vi "Intellirupter_main.vi"() -> ()   [LabVIEW 2016]
uses:
  <vilib>/Platform/TimedLoop/XDataNode/timing_clust.ctl
  <vilib>/Platform/TimedLoop/XDataNode/nitl_modes.ctl
  <vilib>/Platform/TimedLoop/XDataNode/wakeup.ctl
  <vilib>/FPGAPlugInAG/cRIO-9039 (Sync)/niLvFpga_Open_cRIO-9039 (Sync).vi
  <vilib>/rvi/interface/common/dynamic/niFpgaDynamicAddResources.vi
  <vilib>/Utility/error.llb/Error Cluster From Error Code.vi
  <vilib>/rvi/errors/niLvFpgaAdjustHostInterfaceError.vi
  Communication (Yiwei)/Global communication.vi
  <vilib>/FPGAPlugInAG/Dynamic/niLvFpga_Close_Dynamic.vi
  <vilib>/rvi/interface/nirviOpenFPGA/nirviOpenFPGA.xnode
  FPGA Bitfiles/IntelliRupter_calibrated.lvbitx
  <vilib>/rvi/interface/nirviReadWriteControl/nirviReadWriteControl.xnode
  <vilib>/Platform/TimedLoop/XDataNode/XDataNode.xnode
  <vilib>/rvi/interface/nirviCloseFPGA/nirviCloseFPGA.xnode
  <vilib>/rvi/interface/Simulation/niFpgaSimulationCallBeginRW.vi
  NiFpgaLv.dll
  <vilib>/Platform/TimedLoop/XDataNode/XDNodeRunTimeDep.lvlib
panel:
  out "Waveform Chart 2":dbl(graph)
  in  "output cluster":cluster{"reinitialize? (F)":bool, "dt (s)":dbl}={"reinitialize? (F)"=FALSE, "dt (s)"=0.001}
  in  "PID gains":T1={"proportional gain (Kc)"=1.0, "integral time (Ti, min)"=0.001, "derivative time (Td, min)"=0.0} {"derivative time (Td, min)" format="%.3f"; "integral time (Ti, min)" format="%.3f"; "proportional gain (Kc)" format="%.3f"}
  in  "y":dbl
  out "Waveform Chart":dbl(graph)
  in  "I offset R2":dbl=-0.06
  in  "I offset R7":dbl
  in  "I offset R3":dbl=-0.12
  out "R8 Transfer":bool
  out "R7 Transfer":bool
  out "R5 Transfer":bool
  out "R4 Transfer":bool
  out "R2 Transfer":bool
  in  "I offset R8":dbl=0.09
  in  "I offset R4":dbl=-0.07
  in  "I offset R6":dbl=0.095
  in  "I offset R5":dbl=0.02
  in  "I offset R1":dbl=-0.12
  in  "R8 Blocking in":bool
  in  "R7 Blocking in":bool
  in  "R6 Blocking in":bool
  in  "R5 Blocking in":bool
  in  "R4 Blocking in":bool
  in  "R3 Blocking in":bool
  in  "R2 Blocking in":bool
  in  "R1 Blocking in":bool
  out "R1 Blocking out":bool[](array[boolean])
  out "R2 Blocking out":bool[](array[boolean])
  out "R3 Blocking out":bool[](array[boolean])
  out "R4 Blocking out":bool[](array[boolean])
  out "R5 Blocking out":bool[](array[boolean])
  out "R6 Blocking out":bool[](array[boolean])
  out "R8 Blocking out":bool[](array[boolean])
  out "R7 Blocking out":bool[](array[boolean])
  out "Relay7 Reclose":bool=TRUE
  out "Relay7 Trip":bool
  out "Relay8 Reclose":bool=TRUE
  out "Relay8 Trip":bool
  out "Relay6 Reclose":bool=TRUE
  out "Relay6 Trip":bool
  out "Relay5 Reclose":bool=TRUE
  out "Relay5 Trip":bool
  out "Relay4 Reclose":bool=TRUE
  out "Relay4 Trip":bool
  out "Relay3 Reclose":bool=TRUE
  out "Relay3 Trip":bool
  out "Relay2 Reclose":bool=TRUE
  out "Relay2 Trip":bool
  out "Relay1 Reclose":bool=TRUE
  out "Relay1 Trip":bool
  in  "Manual Relay Control":bool
  in  "Reset Relay":bool
  out "Loop time":u32=37
  in  "Recloser Settings":T2={"Magnitude Minimum"=0.1, "Magnitude difference level"=0.1, "Frequency difference level"=0.5, "Phase difference level"=10.0}
  out "MGCC_to_relay":bool[](array[boolean])=[TRUE, TRUE, FALSE, TRUE, TRUE, TRUE, TRUE, TRUE]
  in  "Count(ticks)":u32=10000
  in  "RMS minimum\nvalues":cluster{"VRMS values":dbl, "IRMS values":dbl}={"VRMS values"=0.1, "IRMS values"=0.1}
  out "error out":errorcluster
  out "Relay_toMGCC":bool[](array[boolean])=[TRUE, TRUE, FALSE, TRUE, TRUE, TRUE, TRUE, TRUE]
  in  "Reclose Relay8?":bool=TRUE
  out "R8 Data for\ncommunication":dbl[](array[numeric])=[1.0, 1.0717288119606128, 1.0273744109493954, 60.14375742781454, 60.14096390508348, -0.003401189111173153, 0.13142361409120604, 0.0014423221455373873, 0.0, 0.0]
  in  "Reclose Relay7?":bool=TRUE
  out "R7 Data for\ncommunication":dbl[](array[numeric])=[1.0, 1.0189736883003988, 1.0391105774878193, 60.14220400137767, 60.14841362237464, -0.003401275025680661, -0.31916486626176716, -0.003154578866978825, 0.0, 0.0]
  in  "Reclose Relay6?":bool=TRUE
  out "R6 Data for\ncommunication":dbl[](array[numeric])=[1.0, 1.1139535808581806, 1.0329364281545637, 60.147215439773106, 60.14857986423551, -0.003401093650609255, 0.12186050090227488, -0.001429571057703036, 0.0, 0.0]
  in  "Reclose Relay5?":bool=TRUE
  out "R5 Data for\ncommunication":dbl[](array[numeric])=[1.0, 1.1121379065253558, 1.0317589511765997, 60.14737789614628, 60.15040153111249, -0.0034011360257864, -0.20946315978329266, -0.0021582839957721063, 0.0, 0.0]
  in  "Reclose Relay4?":bool=TRUE
  out "R4 Data for\ncommunication":dbl[](array[numeric])=[1.0, 1.0686115234679994, 1.0027287608315838, 60.152969027967806, 60.13754923755685, -0.0034010736271739006, -0.14980308382633703, 0.0013760159412812356, 0.0, 0.0]
  in  "Reclose Relay3?":bool
  out "R3 Data for\ncommunication":dbl[](array[numeric])=[0.0, 1.07782975233832, 0.003387393613972556, 60.14899592139225, 60.0, -0.003399668261408806, -0.0034568490312473234, -0.00019198572190906357, 0.0, 0.0]
  in  "Reclose Relay2?":bool=TRUE
  out "R2 Data for\ncommunication":dbl[](array[numeric])=[1.0, 1.0375425764882493, 1.093816325060775, 60.14953625389711, 60.14380481717145, -0.005668502300977707, -0.07757149977492932, 0.0008310640468781044, 0.0, 0.06200518529818666]
  out "R1 Data for\ncommunication":dbl[](array[numeric])=[1.0, 1.0412221867764977, 1.0835351412036465, 60.14975919726576, 60.14405490254401, -0.0034011071547865868, -0.06774706733438597, 0.0006251405286130218, 0.0, 0.04801724914889416]
  in  "Relay8":bool=TRUE
  in  "Relay7":bool=TRUE
  in  "Relay6":bool=TRUE
  in  "Relay5":bool=TRUE
  in  "Relay4":bool=TRUE
  in  "Relay3":bool
  in  "Relay2":bool=TRUE
  in  "Reclose Relay1?":bool=TRUE
  in  "stop":bool
  in  "Relay1":bool=TRUE
  # "status\nmag_left\nmag_right\nfreq_left\nfreq_right\nang_diff\nact_power\nrea_power\n0\n0"
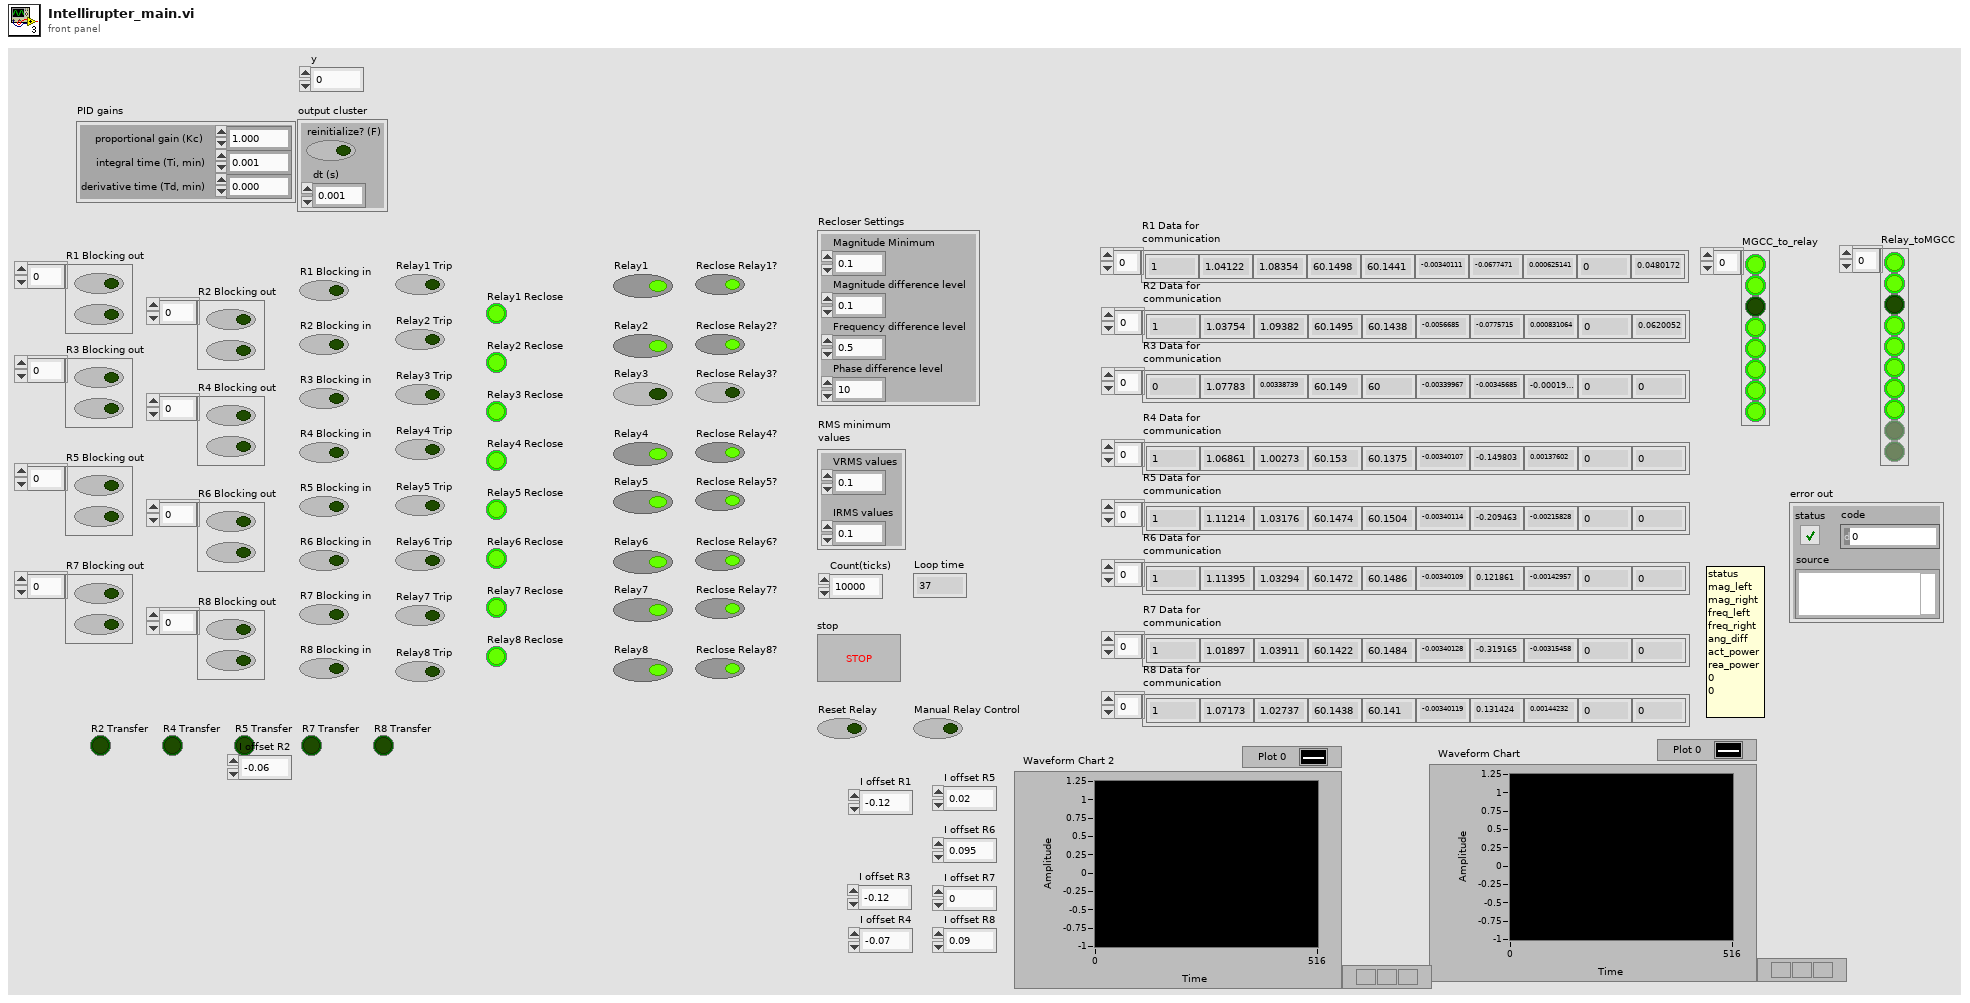
[diagram p1: front panel]
types:
  T1 = cluster{"proportional gain (Kc)":dbl, "integral time (Ti, min)":dbl, "derivative time (Td, min)":dbl}
  T2 = cluster{"Magnitude Minimum":dbl, "Magnitude difference level":dbl, "Frequency difference level":dbl, "Phase difference level":dbl}
  T3 = typedef "XDNodeRunTimeDep.lvlib/timing_clust.ctl" = cluster{"Expected End [f-1]":u64, "Actual End [f-1]":u64, "Finished Late? [f-1]":bool, "Expected End [i-1]":u64, "Actual End [i-1]":u64, "Finished Late? [i-1]":bool, "Expected Start [i]":u64, "Actual Start [i]":u64, "Expected Start [f]":u64, "Actual Start [f]":u64, "Source Name":string, "Structure Name":string, "Period":i64, "Deadline":i64, "Offset":i64, "Start":i64, "Priority":i32, "Timeout":i32, "Mode":T4, "Wakeup Reason":T5, "Error":errorcluster, "Source Type":string, "Secondary Source Type":string, "Global End Time":u64, "Global Start Time":u64, "Frame Duration":u64, "Iteration Duration":u64, "Assigned CPU":i32, "I/O Scan Engine Mode":u32}
  T4 = typedef "XDNodeRunTimeDep.lvlib/nitl_modes.ctl" = enum32{"No Change", "Process missed periods, maintain original phase", "Discard missed periods, maintain original phase", "Process missed periods, ignore original phase", "Discard missed periods, ignore original phase"}
  T5 = typedef "XDNodeRunTimeDep.lvlib/wakeup.ctl" = enum32{"Normal", "Aborted", "Asynchronous wakeup", "Timing source error", "Timed loop error", "Timeout"}
  T6 = cluster{"UV Reset level":dbl, "Undervoltage \npick-up level":dbl, "OC Reset level":dbl, "Overcurrent\npick-up level":dbl, "time delay settings":cluster{"Definite operate time [ms]":u32, "Inverse Operating Time [ms]":u32, "reset time [ms]":u32, "operate time compensation [ms]":u32}}
  T7 = cluster{"V2L AB":fxp<+/-,53,11>, "V2L BC":fxp<+/-,53,11>, "V2L CA":fxp<+/-,53,11>, "V2R AB":fxp<+/-,53,11>, "V2R BC":fxp<+/-,53,11>, "V2R CA":fxp<+/-,53,11>, "I2 A":fxp<+/-,53,11>, "I2 B":fxp<+/-,53,11>, "I2 C":fxp<+/-,53,11>}
  T8 = cluster{"V8L AB":fxp<+/-,53,11>, "V8L BC":fxp<+/-,53,11>, "V8L CA":fxp<+/-,53,11>, "V8R AB":fxp<+/-,53,11>, "V8R BC":fxp<+/-,53,11>, "V8R CA":fxp<+/-,53,11>, "I8 A":fxp<+/-,53,11>, "I8 B":fxp<+/-,53,11>, "I8 C":fxp<+/-,53,11>}
  T9 = cluster{"V7L AB":fxp<+/-,53,11>, "V7L BC":fxp<+/-,53,11>, "V7L CA":fxp<+/-,53,11>, "V7R AB":fxp<+/-,53,11>, "V7R BC":fxp<+/-,53,11>, "V7R CA":fxp<+/-,53,11>, "I7 A":fxp<+/-,53,11>, "I7 B":fxp<+/-,53,11>, "I7 C":fxp<+/-,53,11>}
  T10 = cluster{"V6L AB":fxp<+/-,53,11>, "V6L BC":fxp<+/-,53,11>, "V6L CA":fxp<+/-,53,11>, "V6R AB":fxp<+/-,53,11>, "V6R BC":fxp<+/-,53,11>, "V6R CA":fxp<+/-,53,11>, "I6 A":fxp<+/-,53,11>, "I6 B":fxp<+/-,53,11>, "I6 C":fxp<+/-,53,11>}
  T11 = cluster{"V1L AB":fxp<+/-,53,11>, "V1L BC":fxp<+/-,53,11>, "V1L CA":fxp<+/-,53,11>, "V1R AB":fxp<+/-,53,11>, "V1R BC":fxp<+/-,53,11>, "V1R CA":fxp<+/-,53,11>, "I1 A":fxp<+/-,53,11>, "I1 B":fxp<+/-,53,11>, "I1 C":fxp<+/-,53,11>}
  T12 = cluster{"V3L AB":fxp<+/-,53,11>, "V3L BC":fxp<+/-,53,11>, "V3L CA":fxp<+/-,53,11>, "V3R AB":fxp<+/-,53,11>, "V3R BC":fxp<+/-,53,11>, "V3R CA":fxp<+/-,53,11>, "I3 A":fxp<+/-,53,11>, "I3 B":fxp<+/-,53,11>, "I3 C":fxp<+/-,53,11>}
  T13 = cluster{"V5L AB":fxp<+/-,53,11>, "V5L BC":fxp<+/-,53,11>, "V5L CA":fxp<+/-,53,11>, "V5R AB":fxp<+/-,53,11>, "V5R BC":fxp<+/-,53,11>, "V5R CA":fxp<+/-,53,11>, "I5 A":fxp<+/-,53,11>, "I5 B":fxp<+/-,53,11>, "I5 C":fxp<+/-,53,11>}
  T14 = cluster{"V4L AB":fxp<+/-,53,11>, "V4L BC":fxp<+/-,53,11>, "V4L CA":fxp<+/-,53,11>, "V4R AB":fxp<+/-,53,11>, "V4R BC":fxp<+/-,53,11>, "V4R CA":fxp<+/-,53,11>, "I4 A":fxp<+/-,53,11>, "I4 B":fxp<+/-,53,11>, "I4 C":fxp<+/-,53,11>}
  T15 = typedef "NI_EP_Protection_FPGA.lvlib/fpga_Timer Feedback Var.ctl" = cluster{"time elapsed":u32, "start time of trip counting":u32, "start time of reseting":u32}
  T16 = typedef "NI_EP_Protection_FPGA.lvlib/fpga_State.ctl" = enum16{"Idle", "Trip Counting", "Tripped", "Reset Counting"}
  T17 = cluster{"Direction":enum16{"forward", "backward", "N/D"}, "Boolean":bool, "timing values out":T15, "status out":T16, "trip signal out":bool, "State Out":enum16{"Idle", "Wait for Trip", "PulseClosing", "Locked"}, "Pulse Index Out":i32, "start time of reseting":u32}
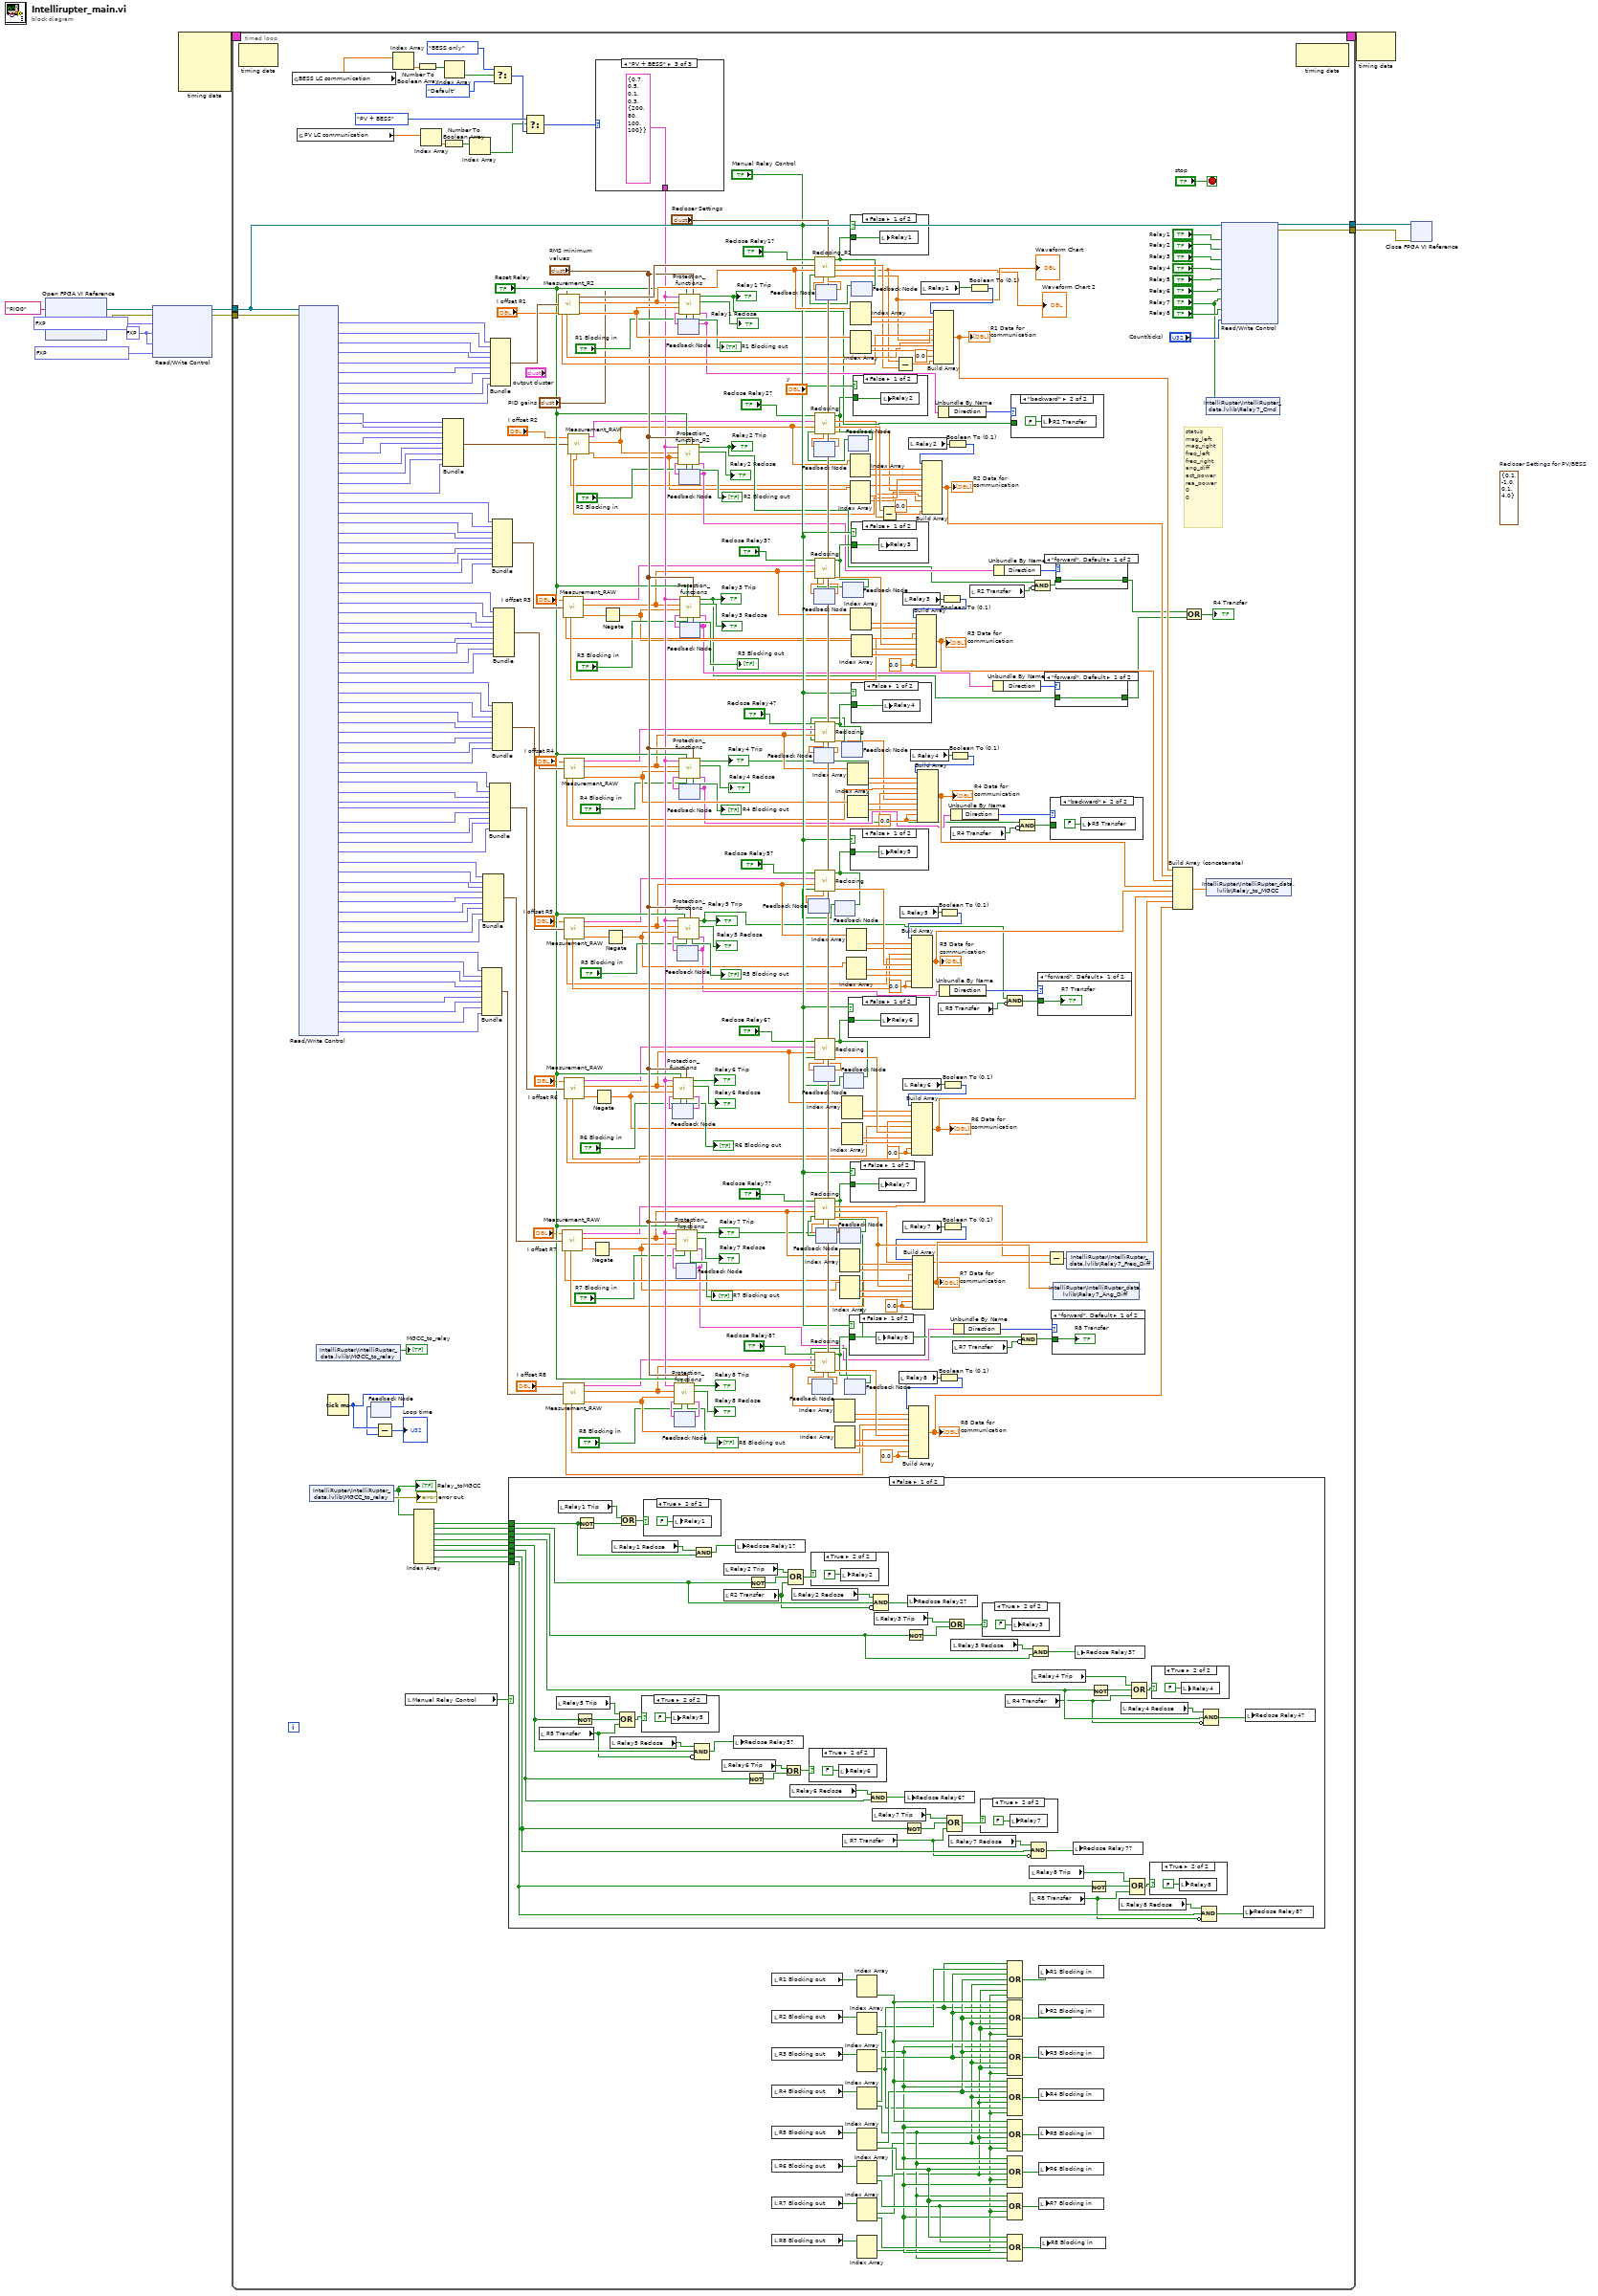
[diagram p0: block diagram]
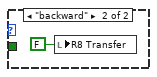
[diagram p2: hidden frame]
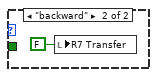
[diagram p3: hidden frame]
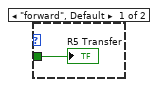
[diagram p4: hidden frame]
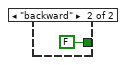
[diagram p5: hidden frame]
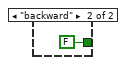
[diagram p6: hidden frame]
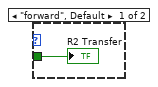
[diagram p7: hidden frame]
diagram:
  (unwired) T2 {"Magnitude Minimum"=0.1, "Magnitude difference level"=-1.0, "Frequency difference level"=0.1, "Phase difference level"=4.0}  # Recloser Settings for PV/BESS
  w4 = fxp<+/-,52,10> 0.0 ("I offset")
  n1 = xnode "Open FPGA VI Reference"("resource name"=tag "RIO0") -> ("FPGA VI Reference Out"=w3:refnum<k20>, "error out"=w8:errorcluster)  [unwired: 1 in]
  n2 = xnode "Read/Write Control"("FPGA VI Reference In"=w3, "error in"=w8, "I scale factor"=fxp<+/-,26,5> 0.4850001335144043, "I offset"=w4, "V offset"=w4, "V scale factor"=fxp<+/-,26,5> 0.40000009536743164) -> ("FPGA VI Reference Out"=w9:refnum<k20>, "error out"=w7:errorcluster)
  n3 = node-c288() -> (w2:T3)  [unwired: 4 in]
  n4 = timed-loop {
    tunnel: w9 -> [w405]
    tunnel: [w407] -> w11
    tunnel: [w406] -> w10
    tunnel: w7 -> [w404]
    timing: w2 -> [_]
    timing-out: [_] -> w1
    stop <- "stop" stop-if-true
    w173 = 0.0 ("element")
    w174 = 0.0 ("element")
    w189 = 0.0 ("element")
    w190 = 0.0 ("element")
    w207 = 0.0 ("element")
    w208 = 0.0 ("element")
    # "status\nmag_left\nmag_right\nfreq_left\nfreq_right\nang_diff\nact_power\nrea_power\n0\n0"
    n5 = node-c288() -> ()  [unwired: 1 in, 1 out]
    n6 = global read "Global communication.vi" "BESS LC communication"() -> (w227:dbl[])
    n7 = global read "Global communication.vi" "PV LC communication"() -> (w226:dbl[])
    n8 = xnode "Read/Write Control"("FPGA VI Reference In"=w405, "error in"=w404) -> ("V1L AB"=w225:fxp<+/-,53,11>, "V1L BC"=w403:fxp<+/-,53,11>, "V1L CA"=w402:fxp<+/-,53,11>, "V1R AB"=w401:fxp<+/-,53,11>, "V1R BC"=w400:fxp<+/-,53,11>, "V1R CA"=w399:fxp<+/-,53,11>, "I1 A"=w398:fxp<+/-,53,11>, "I1 B"=w397:fxp<+/-,53,11>, "I1 C"=w396:fxp<+/-,53,11>, "V2L AB"=w36:fxp<+/-,53,11>, "V2L BC"=w35:fxp<+/-,53,11>, "V2L CA"=w34:fxp<+/-,53,11>, "V2R AB"=w33:fxp<+/-,53,11>, "V2R BC"=w32:fxp<+/-,53,11>, "V2R CA"=w31:fxp<+/-,53,11>, "I2 A"=w30:fxp<+/-,53,11>, "I2 B"=w29:fxp<+/-,53,11>, "I2 C"=w28:fxp<+/-,53,11>, "V3L AB"=w381:fxp<+/-,53,11>, "V3L BC"=w380:fxp<+/-,53,11>, "V3L CA"=w379:fxp<+/-,53,11>, "V3R AB"=w378:fxp<+/-,53,11>, "V3R BC"=w377:fxp<+/-,53,11>, "V3R CA"=w376:fxp<+/-,53,11>, "I3 A"=w375:fxp<+/-,53,11>, "I3 B"=w374:fxp<+/-,53,11>, "I3 C"=w373:fxp<+/-,53,11>, "V4L AB"=w372:fxp<+/-,53,11>, "V4L BC"=w371:fxp<+/-,53,11>, "V4L CA"=w370:fxp<+/-,53,11>, "V4R AB"=w369:fxp<+/-,53,11>, "V4R BC"=w368:fxp<+/-,53,11>, "V4R CA"=w367:fxp<+/-,53,11>, "I4 A"=w366:fxp<+/-,53,11>, "I4 B"=w365:fxp<+/-,53,11>, "I4 C"=w364:fxp<+/-,53,11>, "V5L AB"=w363:fxp<+/-,53,11>, "V5L BC"=w362:fxp<+/-,53,11>, "V5L CA"=w361:fxp<+/-,53,11>, "V5R AB"=w360:fxp<+/-,53,11>, "V5R BC"=w359:fxp<+/-,53,11>, "V5R CA"=w358:fxp<+/-,53,11>, "I5 A"=w357:fxp<+/-,53,11>, "I5 B"=w356:fxp<+/-,53,11>, "I5 C"=w355:fxp<+/-,53,11>, "V6L AB"=w354:fxp<+/-,53,11>, "V6L BC"=w353:fxp<+/-,53,11>, "V6L CA"=w352:fxp<+/-,53,11>, "V6R AB"=w351:fxp<+/-,53,11>, "V6R BC"=w350:fxp<+/-,53,11>, "V6R CA"=w349:fxp<+/-,53,11>, "I6 A"=w348:fxp<+/-,53,11>, "I6 B"=w347:fxp<+/-,53,11>, "I6 C"=w346:fxp<+/-,53,11>, "V7L AB"=w345:fxp<+/-,53,11>, "V7L BC"=w344:fxp<+/-,53,11>, "V7L CA"=w343:fxp<+/-,53,11>, "V7R AB"=w342:fxp<+/-,53,11>, "V7R BC"=w341:fxp<+/-,53,11>, "V7R CA"=w340:fxp<+/-,53,11>, "I7 A"=w339:fxp<+/-,53,11>, "I7 B"=w338:fxp<+/-,53,11>, "I7 C"=w337:fxp<+/-,53,11>, "V8L AB"=w336:fxp<+/-,53,11>, "V8L BC"=w335:fxp<+/-,53,11>, "V8L CA"=w334:fxp<+/-,53,11>, "V8R AB"=w333:fxp<+/-,53,11>, "V8R BC"=w332:fxp<+/-,53,11>, "V8R CA"=w331:fxp<+/-,53,11>, "I8 A"=w330:fxp<+/-,53,11>, "I8 B"=w329:fxp<+/-,53,11>, "I8 C"=w328:fxp<+/-,53,11>)  [unwired: 2 out]
    n9 = shared-variable "IntelliRupter\\IntelliRupter_data.lvlib\\MGCC_to_relay"() -> (w315:bool[], error out=→"error out":errorcluster)  [unwired: 1 in]
    "Relay_toMGCC" <- w315
    n10 = shared-variable "IntelliRupter\\IntelliRupter_data.lvlib\\MGCC_to_relay"() -> (→"MGCC_to_relay":bool[])  [unwired: 1 in, 1 out]
    n11 = Tick Count (ms)() -> (millisecond timer value=w299:u32)
    n12 = feedback #1() -> (w298:u32)  [unwired: 1 in]
    n13 = feedback-in #1(w299) -> ()
    n14 = Subtract(x=w299, y=w298) -> (x-y=→"Loop time":u32)
    n15 = Index Array(array=w227) -> (element=w303:dbl)  [unwired: 1 in]
    n16 = local read "Manual Relay Control"() -> (w274:bool)
    n17 = Index Array(array=w315) -> (element #1=w282:bool, element #2=w281:bool, element #3=w280:bool, element #4=w279:bool, element #5=w278:bool, element #6=w277:bool, element #7=w276:bool, element #8=w275:bool)  [unwired: 8 in]
    n18 = Number To Boolean Array(number=w303) -> (Boolean array=w310:bool[])
    n19 = Index Array(array=w226) -> (element=w306:dbl)  [unwired: 1 in]
    n20 = Bundle("V2L AB"=w36, "V2L BC"=w35, "V2L CA"=w34, "V2R AB"=w33, "V2R BC"=w32, "V2R CA"=w31, "I2 A"=w30, "I2 B"=w29, "I2 C"=w28) -> (w27:T7)  [unwired: 1 in]
    n21 = Number To Boolean Array(number=w306) -> (Boolean array=w305:bool[])
    n22 = Index Array(array=w310) -> (element=w309:bool)  [unwired: 1 in]
    n23 = Index Array(array=w305) -> (element=w304:bool)  [unwired: 1 in]
    n24 = Bundle("V8L AB"=w336, "V8L BC"=w335, "V8L CA"=w334, "V8R AB"=w333, "V8R BC"=w332, "V8R CA"=w331, "I8 A"=w330, "I8 B"=w329, "I8 C"=w328) -> (w291:T8)  [unwired: 1 in]
    n25 = Bundle("V7L AB"=w345, "V7L BC"=w344, "V7L CA"=w343, "V7R AB"=w342, "V7R BC"=w341, "V7R CA"=w340, "I7 A"=w339, "I7 B"=w338, "I7 C"=w337) -> (w292:T9)  [unwired: 1 in]
    n26 = Bundle("V6L AB"=w354, "V6L BC"=w353, "V6L CA"=w352, "V6R AB"=w351, "V6R BC"=w350, "V6R CA"=w349, "I6 A"=w348, "I6 B"=w347, "I6 C"=w346) -> (w293:T10)  [unwired: 1 in]
    n27 = Bundle("V1L AB"=w225, "V1L BC"=w403, "V1L CA"=w402, "V1R AB"=w401, "V1R BC"=w400, "V1R CA"=w399, "I1 A"=w398, "I1 B"=w397, "I1 C"=w396) -> (w395:T11)  [unwired: 1 in]
    n28 = Select(t=enum16{"Default", "BESS only", "PV + BESS"}."BESS only", s=w309, f=enum16{"Default", "BESS only", "PV + BESS"}."Default") -> (s? t:f=w311:enum16{"Default", "BESS only", "PV + BESS"})
    n29 = Bundle("V3L AB"=w381, "V3L BC"=w380, "V3L CA"=w379, "V3R AB"=w378, "V3R BC"=w377, "V3R CA"=w376, "I3 A"=w375, "I3 B"=w374, "I3 C"=w373) -> (w296:T12)  [unwired: 1 in]
    n30 = Bundle("V5L AB"=w363, "V5L BC"=w362, "V5L CA"=w361, "V5R AB"=w360, "V5R BC"=w359, "V5R CA"=w358, "I5 A"=w357, "I5 B"=w356, "I5 C"=w355) -> (w294:T13)  [unwired: 1 in]
    n31 = Bundle("V4L AB"=w372, "V4L BC"=w371, "V4L CA"=w370, "V4R AB"=w369, "V4R BC"=w368, "V4R CA"=w367, "I4 A"=w366, "I4 B"=w365, "I4 C"=w364) -> (w295:T14)  [unwired: 1 in]
    n32 = case shown="False" w274 {
      tunnel: w282 -> [w468 _]
      tunnel: w281 -> [w466 _]
      tunnel: w280 -> [w462 _]
      tunnel: w279 -> [w459 _]
      tunnel: w278 -> [w438 _]
      tunnel: w277 -> [w437 _]
      tunnel: w276 -> [w436 _]
      tunnel: w275 -> [w435 _]
      frame False {
        n33 = local read "R5 Transfer"() -> (w432:bool)
        n34 = local read "Relay5 Trip"() -> (w439:bool)
        n35 = local read "Relay1 Trip"() -> (w482:bool)
        n36 = Not(x=w438) -> (.not. x?=w441:bool)
        n37 = Not(x=w468) -> (.not. x?=w480:bool)
        n38 = local read "Relay5 Reclose"() -> (w452:bool)
        n39 = local read "Relay1 Reclose"() -> (w469:bool)
        n40 = Or(x=w482, y=w480) -> (x .or. y?=w481:bool)
        n41 = Compound Arithmetic op=OR(w439, w441, w432) -> (w440:bool)
        n42 = case shown="True" w440 {
          frame False {
          }
          frame True {
            n43 = local write "Relay5"(FALSE ("Relay8")) -> ()
          }
        }
        n44 = case shown="True" w481 {
          frame False {
          }
          frame True {
            n45 = local write "Relay1"(FALSE ("Relay8")) -> ()
          }
        }
        n46 = And(x=w469, y=w468) -> (x .and. y?=w470:bool)
        n47 = Compound Arithmetic op=AND(w452, w438, invert w432) -> (w451:bool)
        n48 = local read "Relay6 Trip"() -> (w448:bool)
        n49 = local read "Relay2 Trip"() -> (w473:bool)
        n50 = local read "R2 Transfer"() -> (w434:bool)
        n51 = local write "Reclose Relay5?"(w451) -> ()
        n52 = local write "Reclose Relay1?"(w470) -> ()
        n53 = Not(x=w437) -> (.not. x?=w442:bool)
        n54 = Not(x=w466) -> (.not. x?=w479:bool)
        n55 = Or(x=w448, y=w442) -> (x .or. y?=w443:bool)
        n56 = Compound Arithmetic op=OR(w473, w479, w434) -> (w478:bool)
        n57 = local read "Relay6 Reclose"() -> (w454:bool)
        n58 = local read "Relay2 Reclose"() -> (w465:bool)
        n59 = case shown="True" w443 {
          frame False {
          }
          frame True {
            n60 = local write "Relay6"(FALSE ("Relay8")) -> ()
          }
        }
        n61 = case shown="True" w478 {
          frame False {
          }
          frame True {
            n62 = local write "Relay2"(FALSE ("Relay8")) -> ()
          }
        }
        n63 = local read "R7 Transfer"() -> (w431:bool)
        n64 = And(x=w454, y=w437) -> (x .and. y?=w453:bool)
        n65 = local read "Relay7 Trip"() -> (w449:bool)
        n66 = Compound Arithmetic op=AND(w465, w466, invert w434) -> (w467:bool)
        n67 = local read "Relay3 Trip"() -> (w472:bool)
        n68 = Not(x=w436) -> (.not. x?=w445:bool)
        n69 = local write "Reclose Relay6?"(w453) -> ()
        n70 = Not(x=w462) -> (.not. x?=w476:bool)
        n71 = local write "Reclose Relay2?"(w467) -> ()
        n72 = Or(x=w472, y=w476) -> (x .or. y?=w477:bool)
        n73 = Compound Arithmetic op=OR(w449, w445, w431) -> (w444:bool)
        n74 = local read "Relay7 Reclose"() -> (w456:bool)
        n75 = local read "Relay3 Reclose"() -> (w463:bool)
        n76 = case shown="True" w444 {
          frame False {
          }
          frame True {
            n77 = local write "Relay7"(FALSE ("Relay8")) -> ()
          }
        }
        n78 = case shown="True" w477 {
          frame False {
          }
          frame True {
            n79 = local write "Relay3"(FALSE ("Relay8")) -> ()
          }
        }
        n80 = local read "R4 Transfer"() -> (w433:bool)
        n81 = local read "Relay8 Trip"() -> (w450:bool)
        n82 = And(x=w463, y=w462) -> (x .and. y?=w464:bool)
        n83 = local read "R8 Transfer"() -> (w430:bool)
        n84 = Compound Arithmetic op=AND(w456, w436, invert w431) -> (w455:bool)
        n85 = local read "Relay4 Trip"() -> (w471:bool)
        n86 = local write "Reclose Relay7?"(w455) -> ()
        n87 = local write "Reclose Relay3?"(w464) -> ()
        n88 = Not(x=w435) -> (.not. x?=w446:bool)
        n89 = Not(x=w459) -> (.not. x?=w475:bool)
        n90 = local read "Relay8 Reclose"() -> (w457:bool)
        n91 = local read "Relay4 Reclose"() -> (w461:bool)
        n92 = Compound Arithmetic op=OR(w450, w446, w430) -> (w447:bool)
        n93 = Compound Arithmetic op=OR(w471, w475, w433) -> (w474:bool)
        n94 = case shown="True" w447 {
          frame False {
          }
          frame True {
            n95 = local write "Relay8"(FALSE ("Relay8")) -> ()
          }
        }
        n96 = case shown="True" w474 {
          frame False {
          }
          frame True {
            n97 = local write "Relay4"(FALSE ("Relay8")) -> ()
          }
        }
        n98 = Compound Arithmetic op=AND(w457, w435, invert w430) -> (w458:bool)
        n99 = Compound Arithmetic op=AND(w461, w459, invert w433) -> (w460:bool)
        n100 = local write "Reclose Relay8?"(w458) -> ()
        n101 = local write "Reclose Relay4?"(w460) -> ()
      }
      frame True {
      }
    }
    n102 = Select(t=enum16{"Default", "BESS only", "PV + BESS"}."PV + BESS", s=w304, f=w311) -> (s? t:f=w313:enum16{"Default", "BESS only", "PV + BESS"})
    n103 = call "Measurement_R2.vi"("I offset"="I offset R1", "PID gains"="PID gains", "input cluster"=w395) -> ("VR frequency"=w271:dbl, "VL frequency"=w272:dbl, "PLL output"=w290:cluster{dbl, dbl, dbl, dbl}, "RMS values"=w287:dbl[], "Total power values"=w273:dbl[])  [unwired: 1 in]
    n104 = call "Measurement_RAW.vi"("I offset"="I offset R7", "input cluster"=w292) -> ("VR frequency"=w106:dbl, "VL frequency"=w107:dbl, "PLL output"=w149:cluster{dbl, dbl[], dbl, dbl[]}, "RMS values"=w134:dbl[], "Total power values"=w117:dbl[])  [unwired: 1 in, 1 out]
    n105 = call "Measurement_RAW.vi"("I offset"="I offset R3", "input cluster"=w296) -> ("VR frequency"=w114:dbl, "VL frequency"=w115:dbl, "PLL output"=w157:cluster{dbl, dbl[], dbl, dbl[]}, "RMS values"=w143:dbl[], "Total power values"=w120:dbl[])  [unwired: 1 in, 1 out]
    n106 = call "Measurement_RAW.vi"("I offset"="I offset R8", "input cluster"=w291) -> ("VR frequency"=w104:dbl, "VL frequency"=w105:dbl, "PLL output"=w146:cluster{dbl, dbl[], dbl, dbl[]}, "RMS values"=w131:dbl[], "Total power values"=w116:dbl[])  [unwired: 1 in, 1 out]
    n107 = call "Measurement_RAW.vi"("I offset"="I offset R4", "input cluster"=w295) -> ("VR frequency"=w112:dbl, "VL frequency"=w113:dbl, "PLL output"=w155:cluster{dbl, dbl[], dbl, dbl[]}, "RMS values"=w142:dbl[], "Total power values"=w119:dbl[])  [unwired: 1 in, 1 out]
    n108 = call "Measurement_RAW.vi"("I offset"="I offset R5", "input cluster"=w294) -> ("VR frequency"=w110:dbl, "VL frequency"=w111:dbl, "PLL output"=w154:cluster{dbl, dbl[], dbl, dbl[]}, "RMS values"=w76:dbl[], "Total power values"=w75:dbl[])  [unwired: 1 in, 1 out]
    n109 = call "Measurement_RAW.vi"("I offset"="I offset R6", "input cluster"=w293) -> ("VR frequency"=w108:dbl, "VL frequency"=w109:dbl, "PLL output"=w151:cluster{dbl, dbl[], dbl, dbl[]}, "RMS values"=w137:dbl[], "Total power values"=w118:dbl[])  [unwired: 1 in, 1 out]
    n110 = call "Measurement_RAW.vi"("I offset"="I offset R2", "input cluster"=w27) -> ("VR frequency"=w22:dbl, "VL frequency"=w23:dbl, "PLL output"=w16:cluster{dbl, dbl[], dbl, dbl[]}, "RMS values"=w26:dbl[], "Total power values"=w21:dbl[])  [unwired: 1 in, 1 out]
    n111 = Negate(x=w117) -> (-x=w40:dbl[])
    n112 = Negate(x=w118) -> (-x=w41:dbl[])
    n113 = case shown="\"PV + BESS\"" w313 {
      tunnel: [T6 {"UV Reset level"=0.7, "Undervoltage \npick-up level"=0.5, "OC Reset level"=0.1, "Overcurrent\npick-up level"=0.5, "time delay settings"={"Definite operate time [ms]"=200, "Inverse Operating Time [ms]"=80, "reset time [ms]"=100, "operate time compensation [ms]"=100}} ("Protection settings") T6 {"UV Reset level"=0.7, "Undervoltage \npick-up level"=0.5, "OC Reset level"=0.1, "Overcurrent\npick-up level"=0.5, "time delay settings"={"Definite operate time [ms]"=200, "Inverse Operating Time [ms]"=80, "reset time [ms]"=100, "operate time compensation [ms]"=100}} ("Protection settings") T6 {"UV Reset level"=0.7, "Undervoltage \npick-up level"=0.5, "OC Reset level"=0.1, "Overcurrent\npick-up level"=0.3, "time delay settings"={"Definite operate time [ms]"=200, "Inverse Operating Time [ms]"=80, "reset time [ms]"=100, "operate time compensation [ms]"=100}} ("Protection settings")] -> w238
      frame "Default", Default {
      }
      frame "BESS only" {
      }
      frame "PV + BESS" {
      }
    }
    n114 = Negate(x=w120) -> (-x=w64:dbl[])
    n115 = Negate(x=w75) -> (-x=w70:dbl[])
    n116 = feedback #2() -> (w152:T17)  [unwired: 1 in]
    n117 = call "Protection_functions.vi"("RMS minimum\nvalues"="RMS minimum\nvalues", "Blocking in"="R6 Blocking in", "Reset Relay"="Reset Relay", "input cluster"=w152, "Total power values"=w41, "RMS values"=w137, "Protection settings"=w238) -> ("output cluster"=w153:T17, "Reclose"=→"Relay6 Reclose":bool, "trip signal"=→"Relay6 Trip":bool, "Blocking out"=→"R6 Blocking out":bool[])  [unwired: 1 in]
    n118 = feedback-in #2(w153) -> ()
    n119 = feedback #3() -> (w147:T17)  [unwired: 1 in]
    n120 = call "Protection_functions.vi"("RMS minimum\nvalues"="RMS minimum\nvalues", "Blocking in"="R8 Blocking in", "Reset Relay"="Reset Relay", "input cluster"=w147, "Total power values"=w116, "RMS values"=w131, "Protection settings"=w238) -> ("output cluster"=w148:T17, "Reclose"=→"Relay8 Reclose":bool, "trip signal"=→"Relay8 Trip":bool, "Blocking out"=→"R8 Blocking out":bool[])  [unwired: 1 in]
    n121 = feedback-in #3(w148) -> ()
    n122 = feedback #4() -> (w150:T17)  [unwired: 1 in]
    n123 = call "Protection_functions.vi"("RMS minimum\nvalues"="RMS minimum\nvalues", "Blocking in"="R7 Blocking in", "Reset Relay"="Reset Relay", "input cluster"=w150, "Total power values"=w40, "RMS values"=w134, "Protection settings"=w238) -> ("output cluster"=w46:T17, "Reclose"=→"Relay7 Reclose":bool, "trip signal"=w43:bool, "Blocking out"=→"R7 Blocking out":bool[])  [unwired: 1 in]
    "Relay7 Trip" <- w43
    n124 = feedback-in #4(w46) -> ()
    n125 = feedback #5() -> (w74:T17)  [unwired: 1 in]
    n126 = feedback #6() -> (w288:T17)  [unwired: 1 in]
    n127 = call "Protection_functions.vi"("RMS minimum\nvalues"="RMS minimum\nvalues", "Blocking in"="R5 Blocking in", "Reset Relay"="Reset Relay", "input cluster"=w74, "Total power values"=w70, "RMS values"=w76, "Protection settings"=w238) -> ("output cluster"=w47:T17, "Reclose"=→"Relay5 Reclose":bool, "trip signal"=w48:bool, "Blocking out"=→"R5 Blocking out":bool[])  [unwired: 1 in]
    "Relay5 Trip" <- w48
    n128 = feedback-in #5(w47) -> ()
    n129 = call "Protection_functions.vi"("RMS minimum\nvalues"="RMS minimum\nvalues", "Blocking in"="R1 Blocking in", "Reset Relay"="Reset Relay", "input cluster"=w288, "Total power values"=w273, "RMS values"=w287, "Protection settings"=w238) -> ("output cluster"=w237:T17, "Reclose"=→"Relay1 Reclose":bool, "trip signal"=w236:bool, "Blocking out"=→"R1 Blocking out":bool[])  [unwired: 1 in]
    "Relay1 Trip" <- w236
    n130 = feedback-in #6(w237) -> ()
    n131 = feedback #7() -> (w158:T17)  [unwired: 1 in]
    n132 = call "Protection_function_R2.vi"("RMS minimum\nvalues"="RMS minimum\nvalues", "Blocking in"="R2 Blocking in", "Reset Relay"="Reset Relay", "input cluster"=w158, "Total power values"=w21, "RMS values"=w26, "Protection settings"=w238) -> ("output cluster"=w65:T17, "Reclose"=→"Relay2 Reclose":bool, "trip signal"=w62:bool, "Blocking out"=→"R2 Blocking out":bool[])  [unwired: 1 in]
    "Relay2 Trip" <- w62
    n133 = feedback-in #7(w65) -> ()
    n134 = feedback #8() -> (w156:T17)  [unwired: 1 in]
    n135 = call "Protection_functions.vi"("RMS minimum\nvalues"="RMS minimum\nvalues", "Blocking in"="R4 Blocking in", "Reset Relay"="Reset Relay", "input cluster"=w156, "Total power values"=w119, "RMS values"=w142, "Protection settings"=w238) -> ("output cluster"=w56:T17, "Reclose"=→"Relay4 Reclose":bool, "trip signal"=w53:bool, "Blocking out"=→"R4 Blocking out":bool[])  [unwired: 1 in]
    "Relay4 Trip" <- w53
    n136 = feedback-in #8(w56) -> ()
    n137 = feedback #9() -> (w159:T17)  [unwired: 1 in]
    n138 = call "Protection_functions.vi"("RMS minimum\nvalues"="RMS minimum\nvalues", "Blocking in"="R3 Blocking in", "Reset Relay"="Reset Relay", "input cluster"=w159, "Total power values"=w64, "RMS values"=w143, "Protection settings"=w238) -> ("output cluster"=w58:T17, "Reclose"=→"Relay3 Reclose":bool, "trip signal"=w57:bool, "Blocking out"=→"R3 Blocking out":bool[])  [unwired: 1 in]
    "Relay3 Trip" <- w57
    n139 = feedback-in #9(w58) -> ()
    n140 = local read "R1 Blocking out"() -> (w266:bool[])
    n141 = local read "R2 Blocking out"() -> (w265:bool[])
    n142 = local read "R3 Blocking out"() -> (w264:bool[])
    n143 = local read "R4 Blocking out"() -> (w263:bool[])
    n144 = local read "R5 Blocking out"() -> (w262:bool[])
    n145 = local read "R6 Blocking out"() -> (w261:bool[])
    n146 = local read "R7 Blocking out"() -> (w260:bool[])
    n147 = local read "R8 Blocking out"() -> (w259:bool[])
    n148 = feedback #10() -> (w197:dbl)  [unwired: 1 in]
    n149 = feedback #11() -> (w166:dbl)  [unwired: 1 in]
    n150 = feedback #12() -> (w201:dbl)  [unwired: 1 in]
    n151 = feedback #13() -> (w217:dbl)  [unwired: 1 in]
    n152 = feedback #14() -> (w214:dbl)  [unwired: 1 in]
    n153 = feedback #15() -> (w182:dbl)  [unwired: 1 in]
    n154 = feedback #16() -> (w393:dbl)  [unwired: 1 in]
    n155 = feedback #17() -> (w179:dbl)  [unwired: 1 in]
    n156 = Index Array(array=w131) -> (element #1=w129:dbl, element #2=w130:dbl)  [unwired: 2 in]
    n157 = feedback #18() -> (w96:bool)  [unwired: 1 in]
    n158 = call "Reclosing.vi"("Recloser Settings"="Recloser Settings", "Counter In"=w197, "Reclose In"=w96, "RMS values"=w76, "PLL output"=w154, "Reclose?"="Reclose Relay5?") -> ("Phase difference"=w193:dbl, "Recloser action"=w97:bool, "Counter Out"=w198:dbl)  [unwired: 1 in, 2 out]
    n159 = feedback-in #10(w198) -> ()
    n160 = feedback-in #18(w97) -> ()
    n161 = Index Array(array=w116) -> (element #1=w171:dbl, element #2=w172:dbl)  [unwired: 2 in]
    n162 = Index Array(array=w134) -> (element #1=w133:dbl, element #2=w132:dbl)  [unwired: 2 in]
    n163 = Index Array(array=w40) -> (element #1=w164:dbl, element #2=w175:dbl)  [unwired: 2 in]
    n164 = feedback #19() -> (w92:bool)  [unwired: 1 in]
    n165 = call "Reclosing.vi"("Recloser Settings"="Recloser Settings", "Counter In"=w179, "Reclose In"=w92, "RMS values"=w134, "PLL output"=w149, "Reclose?"="Reclose Relay7?") -> ("Phase difference"=w224:dbl, "frequency difference"=w222:dbl, "magnitude difference"=w223:dbl, "Recloser action"=w93:bool, "Counter Out"=w180:dbl)  [unwired: 1 in]
    n166 = feedback-in #17(w180) -> ()
    n167 = feedback-in #19(w93) -> ()
    n168 = feedback #20() -> (w98:bool)  [unwired: 1 in]
    n169 = call "Reclosing.vi"("Recloser Settings"="Recloser Settings", "Counter In"=w201, "Reclose In"=w98, "RMS values"=w142, "PLL output"=w155, "Reclose?"="Reclose Relay4?") -> ("Phase difference"=w18:dbl, "Recloser action"=w99:bool, "Counter Out"=w200:dbl)  [unwired: 1 in, 2 out]
    n170 = feedback-in #12(w200) -> ()
    n171 = feedback-in #20(w99) -> ()
    n172 = Index Array(array=w137) -> (element #1=w136:dbl, element #2=w135:dbl)  [unwired: 2 in]
    n173 = Index Array(array=w41) -> (element #1=w187:dbl, element #2=w188:dbl)  [unwired: 2 in]
    n174 = feedback #21() -> (w100:bool)  [unwired: 1 in]
    n175 = call "Reclosing.vi"("Recloser Settings"="Recloser Settings", "Counter In"=w214, "Reclose In"=w100, "RMS values"=w143, "PLL output"=w157, "Reclose?"="Reclose Relay3?") -> ("Phase difference"=w210:dbl, "Recloser action"=w101:bool, "Counter Out"=w215:dbl)  [unwired: 1 in, 2 out]
    n176 = feedback-in #14(w215) -> ()
    n177 = feedback-in #21(w101) -> ()
    n178 = feedback #22() -> (w94:bool)  [unwired: 1 in]
    n179 = call "Reclosing.vi"("Recloser Settings"="Recloser Settings", "Counter In"=w182, "Reclose In"=w94, "RMS values"=w137, "PLL output"=w151, "Reclose?"="Reclose Relay6?") -> ("Phase difference"=w186:dbl, "Recloser action"=w95:bool, "Counter Out"=w181:dbl)  [unwired: 1 in, 2 out]
    n180 = feedback-in #15(w181) -> ()
    n181 = feedback-in #22(w95) -> ()
    n182 = feedback #23() -> (w90:bool)  [unwired: 1 in]
    n183 = call "Reclosing.vi"("Recloser Settings"="Recloser Settings", "Counter In"=w166, "Reclose In"=w90, "RMS values"=w131, "PLL output"=w146, "Reclose?"="Reclose Relay8?") -> ("Phase difference"=w170:dbl, "Recloser action"=w91:bool, "Counter Out"=w165:dbl)  [unwired: 1 in, 2 out]
    n184 = feedback-in #11(w165) -> ()
    n185 = feedback-in #23(w91) -> ()
    n186 = Index Array(array=w76) -> (element #1=w139:dbl, element #2=w138:dbl)  [unwired: 2 in]
    n187 = Index Array(array=w70) -> (element #1=w192:dbl, element #2=w191:dbl)  [unwired: 2 in]
    n188 = Index Array(array=w142) -> (element #1=w141:dbl, element #2=w140:dbl)  [unwired: 2 in]
    n189 = Index Array(array=w119) -> (element #1=w205:dbl, element #2=w206:dbl)  [unwired: 2 in]
    n190 = feedback #24() -> (w102:bool)  [unwired: 1 in]
    n191 = call "Reclosing.vi"("Recloser Settings"="Recloser Settings", "Counter In"=w217, "Reclose In"=w102, "RMS values"=w26, "PLL output"=w16, "Reclose?"="Reclose Relay2?") -> ("Phase difference"=w17:dbl, "frequency difference"=w161:dbl, "magnitude difference"=w160:dbl, "Recloser action"=w103:bool, "Counter Out"=w216:dbl)  [unwired: 1 in]
    n192 = feedback-in #13(w216) -> ()
    n193 = feedback-in #24(w103) -> ()
    n194 = case shown="False" "Manual Relay Control" {
      tunnel: w95 -> [w425 _]
      frame False {
        n195 = local write "Relay6"(w425) -> ()
      }
      frame True {
      }
    }
    n196 = case shown="False" "Manual Relay Control" {
      tunnel: w91 -> [w423 _]
      frame False {
        n197 = local write "Relay8"(w423) -> ()
      }
      frame True {
      }
    }
    n198 = Index Array(array=w26) -> (element #1=w25:dbl, element #2=w24:dbl)  [unwired: 2 in]
    n199 = Index Array(array=w21) -> (element #1=w20:dbl, element #2=w19:dbl)  [unwired: 2 in]
    n200 = case shown="False" "Manual Relay Control" {
      tunnel: w97 -> [w426 _]
      frame False {
        n201 = local write "Relay5"(w426) -> ()
      }
      frame True {
      }
    }
    n202 = case shown="False" "Manual Relay Control" {
      tunnel: w93 -> [w424 _]
      frame False {
        n203 = local write "Relay7"(w424) -> ()
      }
      frame True {
      }
    }
    n204 = Index Array(array=w287) -> (element #1=w286:dbl, element #2=w285:dbl)  [unwired: 2 in]
    n205 = Index Array(array=w273) -> (element #1=w297:dbl, element #2=w389:dbl)  [unwired: 2 in]
    n206 = Index Array(array=w143) -> (element #1=w145:dbl, element #2=w144:dbl)  [unwired: 2 in]
    n207 = feedback #25() -> (w268:bool)  [unwired: 1 in]
    n208 = call "Reclosing_R2.vi"("Recloser Settings"="Recloser Settings", "Counter In"=w393, "Reclose In"=w268, "RMS values"=w287, "PLL output"=w290, "Reclose?"="Reclose Relay1?") -> ("Phase difference"=w14:dbl, "frequency difference"=w13:dbl, "magnitude difference"=w270:dbl, "Recloser action"=w269:bool, "Counter Out"=w394:dbl)  [unwired: 1 in]
    "Waveform Chart" <- w14
    "Waveform Chart 2" <- w13
    n209 = feedback-in #16(w394) -> ()
    n210 = case shown="False" "Manual Relay Control" {
      tunnel: w269 -> [w491 _]
      frame False {
        n211 = local write "Relay1"(w491) -> ()
      }
      frame True {
      }
    }
    n212 = feedback-in #25(w269) -> ()
    n213 = case shown="False" "Manual Relay Control" {
      tunnel: w101 -> [w428 _]
      frame False {
        n214 = local write "Relay3"(w428) -> ()
      }
      frame True {
      }
    }
    n215 = Index Array(array=w64) -> (element #1=w199:dbl, element #2=w209:dbl)  [unwired: 2 in]
    n216 = case shown="False" "Manual Relay Control" {
      tunnel: w99 -> [w427 _]
      frame False {
        n217 = local write "Relay4"(w427) -> ()
      }
      frame True {
      }
    }
    n218 = case shown="False" "Manual Relay Control" {
      tunnel: w103 -> [w429 _]
      frame False {
        n219 = local write "Relay2"(w429) -> ()
      }
      frame True {
      }
    }
    n220 = Index Array(array=w266) -> (element #2=w257:bool)  [unwired: 2 in, 1 out]
    n221 = Index Array(array=w265) -> (element #1=w251:bool, element #2=w232:bool)  [unwired: 2 in]
    n222 = Index Array(array=w264) -> (element #2=w250:bool)  [unwired: 2 in, 1 out]
    n223 = Index Array(array=w263) -> (element #1=w253:bool, element #2=w231:bool)  [unwired: 2 in]
    n224 = Index Array(array=w262) -> (element #1=w252:bool, element #2=w256:bool)  [unwired: 2 in]
    n225 = Index Array(array=w261) -> (element #1=w230:bool, element #2=w255:bool)  [unwired: 2 in]
    n226 = Index Array(array=w260) -> (element #1=w229:bool, element #2=w254:bool)  [unwired: 2 in]
    n227 = Index Array(array=w259) -> (element #1=w228:bool)  [unwired: 2 in, 1 out]
    n228 = Subtract(x=w161, y=w160) -> (x-y=w162:dbl)
    n229 = Subtract(x=w13, y=w270) -> (x-y=w300:dbl)
    n230 = local read "Relay8"() -> (w168:bool)
    n231 = local read "Relay5"() -> (w195:bool)
    n232 = local read "Relay3"() -> (w212:bool)
    n233 = local read "Relay6"() -> (w184:bool)
    n234 = local read "Relay7"() -> (w177:bool)
    n235 = local read "Relay2"() -> (w219:bool)
    n236 = local read "Relay4"() -> (w203:bool)
    n237 = local read "Relay1"() -> (w391:bool)
    n238 = Unbundle By Name(w237) -> ("Direction"=w66:enum16{"forward", "backward", "N/D"})
    n239 = local read "R5 Transfer"() -> (w49:bool)
    n240 = Boolean To (0,1)(Boolean=w168) -> (0, 1=w169:i16)
    n241 = Build Array(w169, w129, w130, w105, w104, w170, w171, w172, w173, w173) -> (w319:dbl[])
    "R8 Data for\ncommunication" <- w319
    n242 = Boolean To (0,1)(Boolean=w195) -> (0, 1=w194:i16)
    n243 = Build Array(w194, w139, w138, w111, w110, w193, w192, w191, w190, w190) -> (w322:dbl[])
    "R5 Data for\ncommunication" <- w322
    n244 = Unbundle By Name(w47) -> ("Direction"=w50:enum16{"forward", "backward", "N/D"})
    n245 = Boolean To (0,1)(Boolean=w212) -> (0, 1=w211:i16)
    n246 = Build Array(w211, w145, w144, w115, w114, w210, w199, w209, w208, w208) -> (w324:dbl[])
    "R3 Data for\ncommunication" <- w324
    n247 = Boolean To (0,1)(Boolean=w184) -> (0, 1=w185:i16)
    n248 = Build Array(w185, w136, w135, w109, w108, w186, w187, w188, w189, w189) -> (w321:dbl[])
    "R6 Data for\ncommunication" <- w321
    n249 = Boolean To (0,1)(Boolean=w177) -> (0, 1=w176:i16)
    n250 = Build Array(w176, w133, w132, w107, w106, w224, w164, w175, w174, w174) -> (w320:dbl[])
    "R7 Data for\ncommunication" <- w320
    n251 = Boolean To (0,1)(Boolean=w219) -> (0, 1=w220:i16)
    n252 = Build Array(w220, w25, w24, w23, w22, w17, w20, w19, 0.0 ("element"), w162) -> (w325:dbl[])
    "R2 Data for\ncommunication" <- w325
    n253 = Boolean To (0,1)(Boolean=w203) -> (0, 1=w204:i16)
    n254 = Build Array(w204, w141, w140, w113, w112, w18, w205, w206, w207, w207) -> (w323:dbl[])
    "R4 Data for\ncommunication" <- w323
    n255 = local read "R4 Transfer"() -> (w52:bool)
    n256 = Unbundle By Name(w56) -> ("Direction"=w55:enum16{"forward", "backward", "N/D"})
    n257 = local read "R7 Transfer"() -> (w44:bool)
    n258 = Unbundle By Name(w46) -> ("Direction"=w45:enum16{"forward", "backward", "N/D"})
    n259 = Boolean To (0,1)(Boolean=w391) -> (0, 1=w390:i16)
    n260 = Build Array(w390, w286, w285, w272, w271, w14, w297, w389, 0.0 ("element"), w300) -> (w326:dbl[])
    "R1 Data for\ncommunication" <- w326
    n261 = local read "R2 Transfer"() -> (w61:bool)
    n262 = Unbundle By Name(w58) -> ("Direction"=w59:enum16{"forward", "backward", "N/D"})
    n263 = Unbundle By Name(w65) -> ("Direction"=w63:enum16{"forward", "backward", "N/D"})
    n264 = Compound Arithmetic op=AND(w48, invert w49) -> (w51:bool)
    n265 = Compound Arithmetic op=OR(w250, w251, w253, w252, w230, w229, w228) -> (w249:bool)
    n266 = Compound Arithmetic op=OR(w257, w250, w253, w252, w230, w229, w228) -> (w248:bool)
    n267 = Compound Arithmetic op=OR(w257, w232, w252, w253, w230, w229, w228) -> (w247:bool)
    n268 = Compound Arithmetic op=OR(w257, w232, w252, w230, w229, w250, w228) -> (w246:bool)
    n269 = Compound Arithmetic op=OR(w257, w232, w231, w229, w230, w228) -> (w245:bool)
    n270 = Compound Arithmetic op=OR(w232, w231, w256, w229, w228, w232) -> (w244:bool)
    n271 = Compound Arithmetic op=OR(w231, w256, w255, w228, w232) -> (w243:bool)
    n272 = Compound Arithmetic op=OR(w256, w255, w254, w232, w231) -> (w242:bool)
    n273 = case shown="\"backward\"" w66 {
      tunnel: w236 -> [w421 _]
      frame "forward", Default {
        "R2 Transfer" <- w421
      }
      frame "backward" {
        n274 = local write "R2 Transfer"(FALSE ("R2 Transfer")) -> ()
      }
    }
    n275 = Compound Arithmetic op=AND(w53, invert w52) -> (w54:bool)
    n276 = Compound Arithmetic op=AND(w43, invert w44) -> (w42:bool)
    n277 = Compound Arithmetic op=AND(w62, invert w61) -> (w60:bool)
    n278 = case shown="\"forward\", Default" w50 {
      tunnel: w51 -> [w413 _]
      frame "forward", Default {
        "R7 Transfer" <- w413
      }
      frame "backward" {
        n279 = local write "R7 Transfer"(FALSE ("R2 Transfer")) -> ()
      }
    }
    n280 = local write "R1 Blocking in"(w249) -> ()
    n281 = local write "R2 Blocking in"(w248) -> ()
    n282 = local write "R3 Blocking in"(w247) -> ()
    n283 = local write "R4 Blocking in"(w246) -> ()
    n284 = local write "R5 Blocking in"(w245) -> ()
    n285 = local write "R6 Blocking in"(w244) -> ()
    n286 = local write "R7 Blocking in"(w243) -> ()
    n287 = local write "R8 Blocking in"(w242) -> ()
    n288 = Subtract(x=w223, y=w222) -> (x-y=w221:dbl)
    n289 = case shown="\"backward\"" w55 {
      tunnel: w54 -> [w415 _]
      frame "forward", Default {
        "R5 Transfer" <- w415
      }
      frame "backward" {
        n290 = local write "R5 Transfer"(FALSE ("R2 Transfer")) -> ()
      }
    }
    n291 = case shown="\"forward\", Default" w45 {
      tunnel: w42 -> [w411 _]
      frame "forward", Default {
        "R8 Transfer" <- w411
      }
      frame "backward" {
        n292 = local write "R8 Transfer"(FALSE ("R2 Transfer")) -> ()
      }
    }
    n293 = shared-variable "IntelliRupter\\IntelliRupter_data.lvlib\\Relay7_Ang_Diff"(w224) -> ()  [unwired: 1 in, 1 out]
    n294 = case shown="\"forward\", Default" w59 {
      tunnel: w57 -> [w417 _]
      tunnel: [w417 FALSE] -> w234
      frame "forward", Default {
      }
      frame "backward" {
      }
    }
    n295 = case shown="\"forward\", Default" w63 {
      tunnel: w60 -> [w419 _]
      tunnel: [w419 FALSE] -> w235
      frame "forward", Default {
      }
      frame "backward" {
      }
    }
    n296 = shared-variable "IntelliRupter\\IntelliRupter_data.lvlib\\Relay7_Freq_Diff"(w221) -> ()  [unwired: 1 in, 1 out]
    n297 = Build Array (concatenate)(w326, w325, w324, w323, w322, w321, w320, w319) -> (w327:dbl[])
    n298 = Or(x=w235, y=w234) -> (x .or. y?=→"R4 Transfer":bool)
    n299 = shared-variable "IntelliRupter\\IntelliRupter_data.lvlib\\Relay_to_MGCC"(w327) -> ()  [unwired: 1 in, 1 out]
    n300 = shared-variable "IntelliRupter\\IntelliRupter_data.lvlib\\Relay7_Cmd"("Relay7") -> ()  [unwired: 1 in, 1 out]
    n301 = xnode "Read/Write Control"("FPGA VI Reference In"=w405, "Relay1"="Relay1", "Relay2"="Relay2", "Relay3"="Relay3", "Relay4"="Relay4", "Relay5"="Relay5", "Relay6"="Relay6", "Relay7"="Relay7", "Relay8"="Relay8", "Count(ticks)"="Count(ticks)") -> ("FPGA VI Reference Out"=w407:refnum<k20>, "error out"=w406:errorcluster)  [unwired: 1 in]
    n302 = node-c288() -> ()  [unwired: 1 in, 1 out]
  }
  n303 = node-c288(w1) -> ()  [unwired: 1 out]
  n304 = xnode "Close FPGA VI Reference"("FPGA VI Reference In"=w11, "error in"=w10) -> ()  [unwired: 1 out]
